vi "Register.vi"(6 "Options":string, 7 "Time out (-1)":i32=-1, 8 "Error in":errorcluster, 9 "INVOCATION event":refnum<user-event>, 10 "Procedure URI":string, 11 "WAMP Client in":refnum<class "WAMP Client.lvclass">) -> (0 "Error out":errorcluster, 2 "Success?":bool, 3 "WAMP Client out":refnum<class "WAMP Client.lvclass">, 5 "WAMP Error":T1={"Details"="{}", "ArgumentKw Payload"="", "Error?"=FALSE, "Error URI"="", "Arguments Payload"=""})   [LabVIEW 2020, in "wamplv.lvlib" / "WAMP Client.lvclass"]
uses:
  WAMP Client.lvclass
  TypeDefs/WAMP error.ctl
  TypeDefs/INVOCATION payload.ctl
  <vilib>/Utility/error.llb/Error Cluster From Error Code.vi
  <vilib>/ErrorRing/Error Ring.xnode
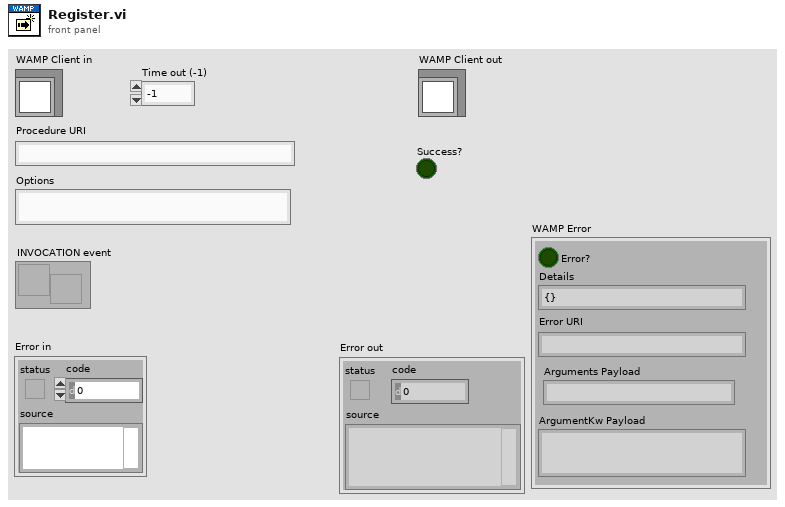
[diagram p1: front panel]
types:
  T1 = typedef "wamplv.lvlib/WAMP Client.lvclass/WAMP error.ctl" = cluster{"Details":string, "ArgumentKw Payload":string, "Error?":bool, "Error URI":string, "Arguments Payload":string}
  T2 = typedef "wamplv.lvlib/WAMP Client.lvclass/Success or error.ctl" = cluster{"Success?":bool, "URI":string, "Combined Error":T3}
  T3 = typedef "wamplv.lvlib/WAMP Client.lvclass/Combined error.ctl" = cluster{"Error?":bool, "WAMP Error":T1, "Error":errorcluster}
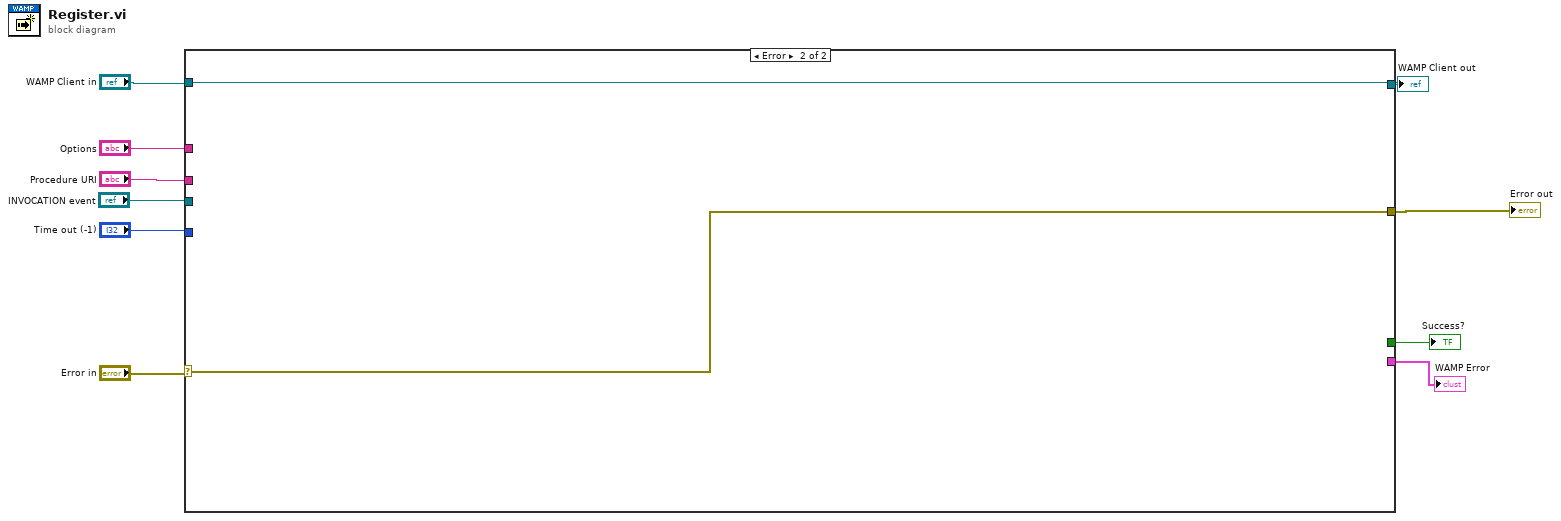
[diagram p0: block diagram]
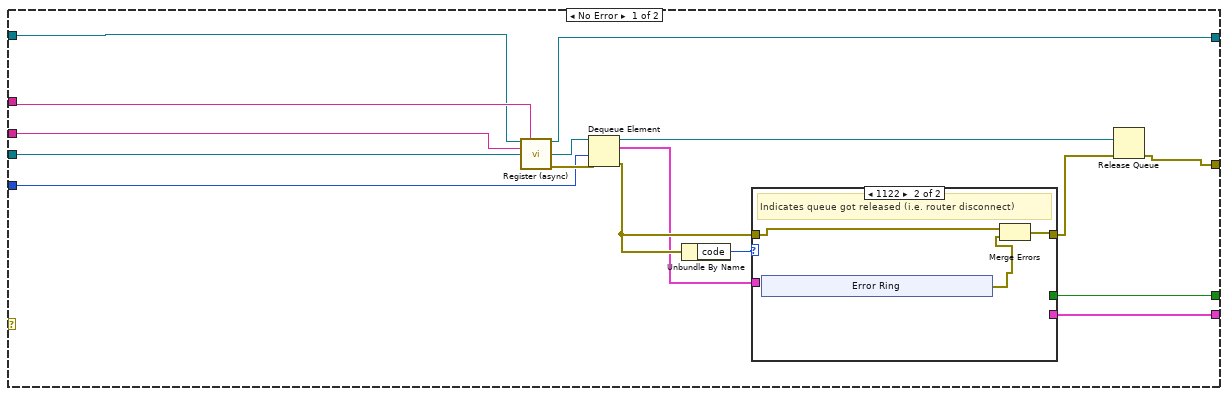
[diagram p2: hidden frame]
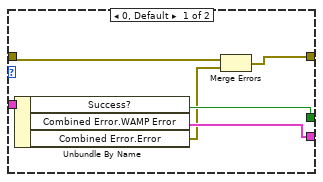
[diagram p3: hidden frame]
diagram:
  n1 = case shown="Error" "Error in" {
    selector: "Error in" -> [_ w41]
    tunnel: [w11 w41] -> w4
    tunnel: [w24 w40] -> w8
    tunnel: "WAMP Client in" -> [w22 w40]
    tunnel: "Procedure URI" -> [w26 _]
    tunnel: "Options" -> [w25 _]
    tunnel: "INVOCATION event" -> [w23 _]
    tunnel: "Time out (-1)" -> [w15 _]
    tunnel: [w14 _] -> w2
    tunnel: [w13 _] -> w1
    frame No Error {
      n2 = call-dynamic "Register (async).vi"("WAMP Client in"=w22, "Options"=w25, "Procedure URI"=w26, "INVOCATION event"=w23) -> ("WAMP Client out"=w24:refnum<class "WAMP Client.lvclass">, "queue out"=w20:refnum<queue>, "error out"=w21:errorcluster)  [unwired: 9 in]
      n3 = Dequeue Element(queue=w20, timeout in ms (-1)=w15, error in (no error)=w21) -> (queue out=w19:refnum<queue>, element=w16:T2, error out=w17:errorcluster)  [unwired: 1 out]
      n4 = Unbundle By Name(w17) -> ("code"=w18:i32)
      n5 = case shown="1122" w18 {
        tunnel: [w29 w35] -> w12
        tunnel: w17 -> [w28 w34]
        tunnel: w16 -> [w32 _]
        tunnel: [w31 _] -> w14
        tunnel: [w30 _] -> w13
        frame 0, Default {
          n6 = Unbundle By Name(w32) -> ("Success?"=w31:bool, "Combined Error.WAMP Error"=w30:T1, "Combined Error.Error"=w27:errorcluster)
          n7 = Merge Errors(w28, w27) -> (w29:errorcluster)
        }
        frame 1122 {
          # "Indicates queue got released (i.e. router disconnect)"
          n8 = xnode "Error Ring"() -> ("error out"=w33:errorcluster)
          n9 = Merge Errors(w34, w33) -> (w35:errorcluster)
        }
      }
      n10 = Release Queue(queue=w19, error in (no error)=w12) -> (error out=w11:errorcluster)  [unwired: 1 in, 2 out]
    }
    frame Error {
    }
  }
  "Error out" <- w4
  "WAMP Client out" <- w8
  "Success?" <- w2
  "WAMP Error" <- w1
